vi "_session_check_list.vi"(7 "VISA resource names in":refnum<visa-resource-name>[](array[refnum]), 8 "error in":errorcluster caption="error in (no error)", 10 "Error if not found (T)":bool=TRUE, 11 "VISA resource name":refnum<visa-resource-name>) -> (0 "error out":errorcluster, 2 "Found in the list":bool, 3 "Session list index out":i32)   [LabVIEW 2022 SP3, in "hmp4000_rsidr_core.lvlib"]
uses:
  hmp4000_rsidr_core.lvlib
  type_Error_Codes.ctl
  Trim Whitespace One-Sided.vi
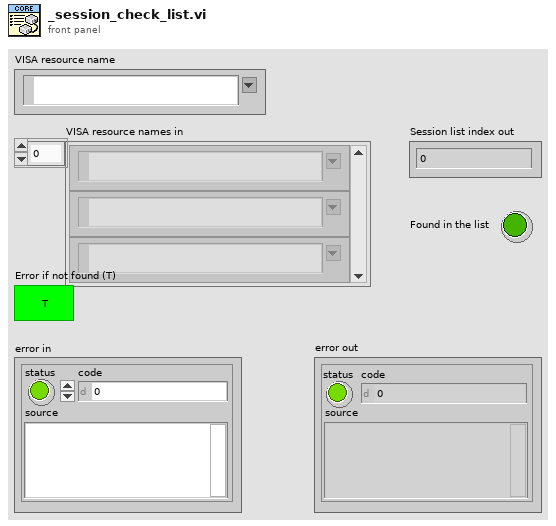
[diagram p1: front panel]
types:
  T1 = typedef "hmp4000_rsidr_core.lvlib/type_Error_Codes.ctl" = enum16{"No_error", "VISA_err_ResourceNotFound", "VISA_err_Timeout", "VISA_warn_MoreDataAvailable", "RS_err_MissingCallback", "RS_err_InvalidAttribute", "RS_err_InvalidValue", "RS_err_UnknownResource", "RS_err_AlreadyInitialized", "RS_err_InstrumentStatus", "RS_err_BadRepCapName", "RS_err_TypesMismatch", "RS_err_ValueNotSupported", "RS_err_InvalidRngTable", "RS_err_IDqueryFail", "RS_err_UnexpResponse", "VISA_warn_ConfigNotLoaded", "RS_err_AttributeNotReadable", "RS_err_AttributeNotWritable", "RS_err_InstrumentType", "RS_err_InstrumentOption", "VISA_err_InvalidSize", "RS_err_ReliabilityIndicator", "VISA_warn_UnknownStatus", "VISA_warn_TermCharRead", "VISA_err_IO_error", "RS_err_FunctionNotSupported", "VISA_warn_QueueEmpty"}
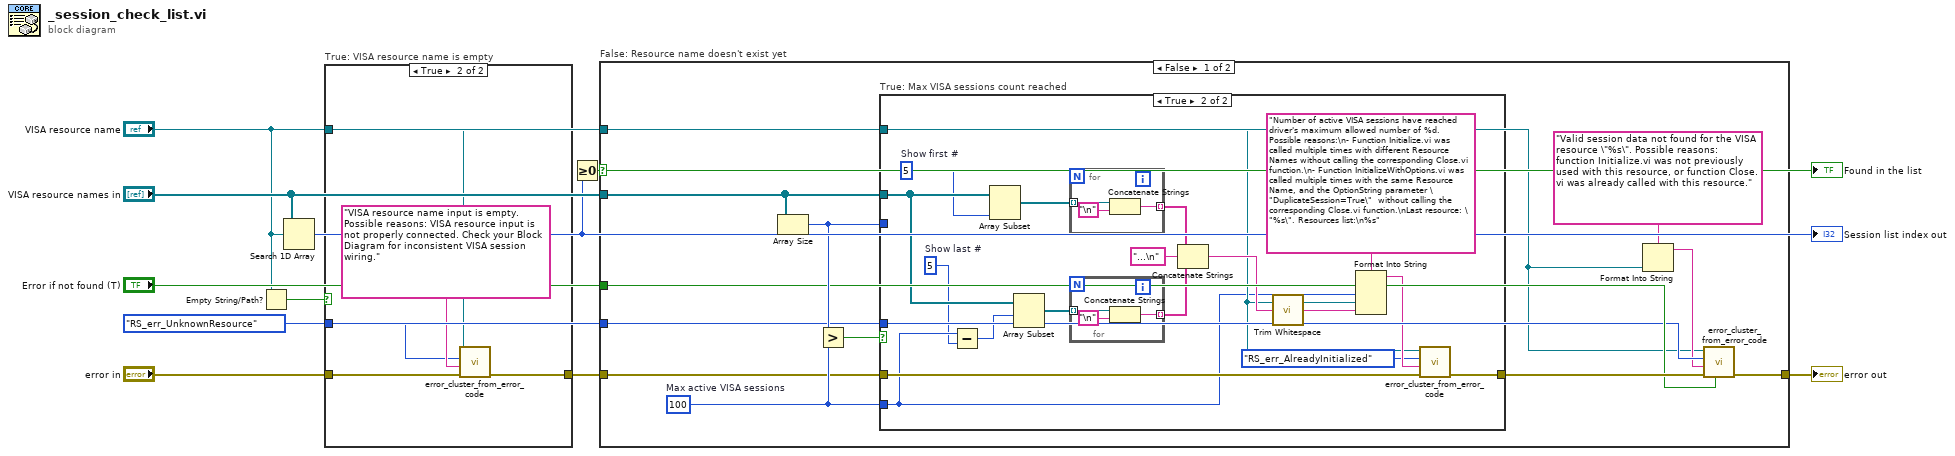
[diagram p0: block diagram]
diagram:
  w2 = type_Error_Codes."RS_err_UnknownResource" ("Error Enum in")
  n1 = Empty String/Path?(string/path="VISA resource name") -> (empty?=w5:bool)
  n2 = Search 1D Array(1D array="VISA resource names in", element="VISA resource name") -> (index of element=w6:i32)  [unwired: 1 in]
  "Session list index out" <- w6
  n3 = case "True: VISA resource name is empty" shown="True" w5 {
    tunnel: "error in" -> [w11 w15]
    tunnel: [w11 w16] -> w4
    tunnel: w2 -> [_ w13]
    tunnel: "VISA resource name" -> [_ w12]
    frame False {
    }
    frame True {
      n4 = call "error_cluster_from_error_code.vi"("error in"=w15, "Error Message (\"\")"="VISA resource name input is empty. Possible reasons: VISA resource input is not properly connected. Check your Block Diagram for inconsistent VISA session wiring." ("error message (\"\")"), "Error Enum in"=w13, "VISA resource name"=w12) -> ("error out"=w16:errorcluster)  [unwired: 6 in, 1 out]
    }
  }
  n5 = Greater Or Equal To 0?(x=w6) -> (x >= 0?=w8:bool)
  "Found in the list" <- w8
  n6 = case "False: Resource name doesn't exist yet" shown="False" w8 {
    tunnel: w4 -> [w20 w54]
    tunnel: [w23 w54] -> w10
    tunnel: "Error if not found (T)" -> [w22 _]
    tunnel: "VISA resource names in" -> [w27 _]
    tunnel: "VISA resource name" -> [w17 _]
    tunnel: w2 -> [w19 _]
    frame False {
      w21 = 100  # Max active VISA sessions
      n7 = Array Size(array=w27) -> (size(s)=w26:i32)
      n8 = Greater?(x=w26, y=w21) -> (0:w28:bool)
      n9 = case "True: Max VISA sessions count reached" shown="True" w28 {
        tunnel: w20 -> [w29 w47]
        tunnel: w19 -> [_ _]
        tunnel: w21 -> [_ w36]
        tunnel: w17 -> [_ w40]
        tunnel: w27 -> [_ w39]
        tunnel: w26 -> [_ _]
        tunnel: [w29 w43] -> w24
        frame False {
        }
        frame True {
          w35 = 5  # Show last #
          w32 = 5  # Show first #
          n10 = Subtract(x=w36, y=w35) -> (x-y=w31:i32)
          n11 = Array Subset(array=w39, length=w32) -> (w46:refnum<visa-resource-name>[])  [unwired: 1 in]
          n12 = Array Subset(array=w39, index=w31) -> (w34:refnum<visa-resource-name>[])  [unwired: 1 in]
          n13 = for {
            tunnel: w46 -> [w53] mode=indexing
            tunnel: [w51] -> w37 mode=indexing
            n14 = Concatenate Strings(w53, "\n" ("Line Feed Constant")) -> (w51:string)
          }
          n15 = for {
            tunnel: w34 -> [w50] mode=indexing
            tunnel: [w48] -> w33 mode=indexing
            n16 = Concatenate Strings(w50, "\n" ("Line Feed Constant")) -> (w48:string)
          }
          n17 = Concatenate Strings(w37, "...\n", w33) -> (w44:string)
          n18 = call "Trim Whitespace.vi"("string"=w44) -> ("trimmed string"=w30:string)  [unwired: 1 in]
          n19 = Format Into String(format string="Number of active VISA sessions have reached driver's maximum allowed number of %d. Possible reasons:\n- Function Initialize.vi was called multiple times with different Resource Names without calling the corresponding Close.vi function.\n- Function InitializeWithOptions.vi was called multiple times with the same Resource Name, and the OptionString parameter \"DuplicateSession=True\"  without calling the corresponding Close.vi function.\nLast resource: \"%s\". Resources list:\n%s" ("error message (\"\")"), w36, w40, w30) -> (resulting string=w42:string)  [unwired: 2 in, 1 out]
          n20 = call "error_cluster_from_error_code.vi"("error in"=w47, "Error Message (\"\")"=w42, "Error Enum in"=type_Error_Codes."RS_err_AlreadyInitialized", "VISA resource name"=w40) -> ("error out"=w43:errorcluster)  [unwired: 6 in, 1 out]
        }
      }
      n21 = Format Into String(format string="Valid session data not found for the VISA resource \"%s\". Possible reasons:  function Initialize.vi was not previously used with this resource, or function Close.vi was already called with this resource." ("error message (\"\")"), w17) -> (resulting string=w18:string)  [unwired: 2 in, 1 out]
      n22 = call "error_cluster_from_error_code.vi"("Error Creation Enabled (True)"=w22, "error in"=w24, "Error Message (\"\")"=w18, "Error Enum in"=w19, "VISA resource name"=w17) -> ("error out"=w23:errorcluster)  [unwired: 5 in, 1 out]
    }
    frame True {
    }
  }
  "error out" <- w10
